vi "Reset Hardware List and Run Button.vi"(8 "error in (no error)":errorcluster, 11 "Measurement UI in":refnum<class "Measurement UI.lvclass">) -> (0 "error out":errorcluster, 3 "Measurement UI out":refnum<class "Measurement UI.lvclass">)   [LabVIEW 2015, in "Measurement UI.lvlib" / "Measurement UI.lvclass"]
uses:
  Measurement UI.lvclass
  Measurement UI.lvclass/Measurement UI.ctl
  Accessors/Read Run.vi
  Accessors/Read Digitizer.vi
  Read Multimeter.vi
  Accessors/Read Function Generator.vi
  Accessors/Read Power Supply.vi
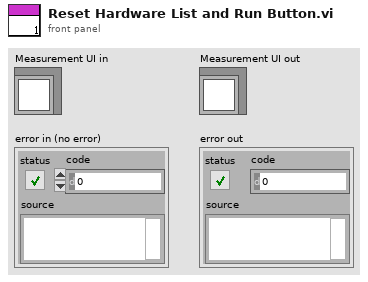
[diagram p1: front panel]
types:
  T1 = enum8{"Enabled", "Disabled", "Disabled and Grayed Out"}
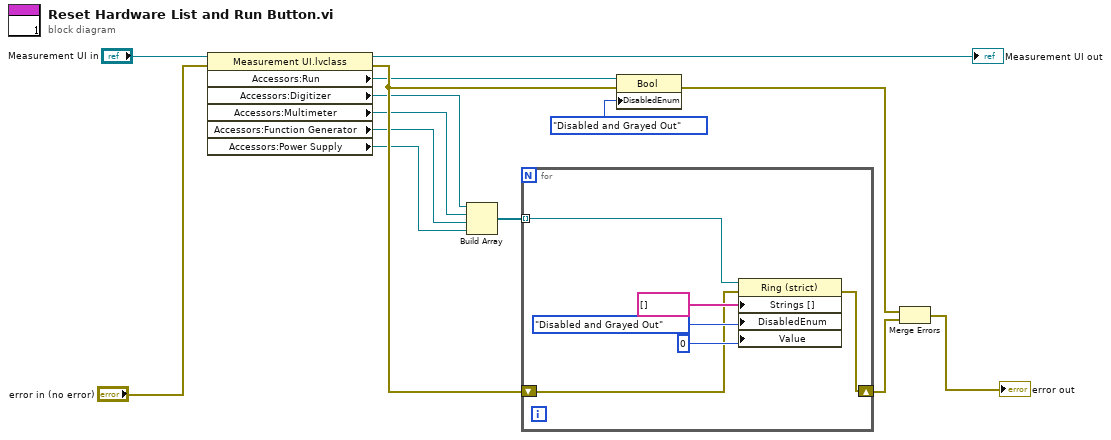
[diagram p0: block diagram]
diagram:
  n1 = property class="Measurement UI.lvclass"(reference="Measurement UI in", error in="error in (no error)") -> (reference out=→"Measurement UI out":refnum<class "Measurement UI.lvclass">, error out=w11:errorcluster, "Accessors:Run"=w10:refnum<vi>, "Accessors:Digitizer"=w4:refnum<vi>, "Accessors:Multimeter"=w5:refnum<vi>, "Accessors:Function Generator"=w6:refnum<vi>, "Accessors:Power Supply"=w7:refnum<vi>)
  n2 = Build Array(w4, w5, w6, w7) -> (w1:refnum<vi>[])
  n3 = for {
    tunnel: w1 -> [w17] mode=indexing
    shift-right: [w16] -> w12
    shift-left: w11 -> [w15]
    n4 = property class="Ring (strict)"(reference=w17, error in=w15, "Strings []"=string[] [], "DisabledEnum"=T1."Disabled and Grayed Out" ("Disabled"), "Value"=u16 0) -> (error out=w16:errorcluster)  [unwired: 1 out]
  }
  n5 = property class="Bool"(reference=w10, error in=w11, "DisabledEnum"=T1."Disabled and Grayed Out" ("Disabled")) -> (error out=w13:errorcluster)  [unwired: 1 out]
  n6 = Merge Errors(w13, w12) -> (→"error out":errorcluster)
